vi "GF_GetAgilentTimeInfo.vi"(8 "error in (no error)":errorcluster, 10 "Timeout (10000 ms)":u32=10000, 11 "VISA resource name":refnum<visa-resource-name>) -> (0 "error out":errorcluster, 2 "Timing Info":cluster{"Name":string, "Value":string}[](array[cluster]), 3 "VISA resource name out":refnum<visa-resource-name>)   [LabVIEW 2020]
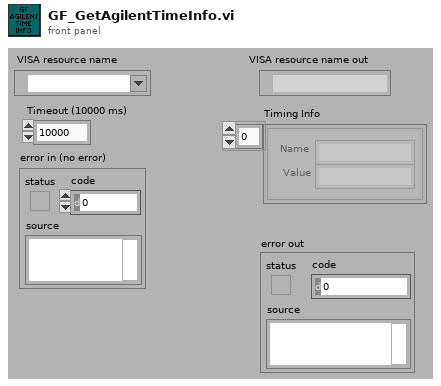
[diagram p1: front panel]
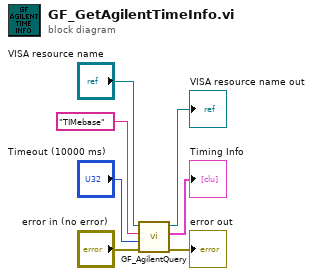
[diagram p0: block diagram]
diagram:
  n1 = call "GF_AgilentQuery.vi"("error in (no error)"="error in (no error)", "Timeout"="Timeout (10000 ms)", "Query"="TIMebase", "Session In"="VISA resource name") -> ("error out"=→"error out":errorcluster, "Token Array 2"=→"Timing Info":cluster{"Name":string, "Value":string}[], "Session out"=→"VISA resource name out":refnum<visa-resource-name>)  [unwired: 4 in]
